vi "SQLite-Modes.vi"   [LabVIEW 2020]
uses:
  <vilib>/drjdpowell/SQLite Library/SQL Statement/SQL Statement.lvclass/SQL Statement.ctl
  <vilib>/drjdpowell/SQLite Library/SQL Connection/Open (path).vi
  <vilib>/drjdpowell/SQLite Library/SQL Statement/Bind Integer.vi
  <vilib>/drjdpowell/SQLite Library/SQL Statement/Bind Real.vi
  <vilib>/drjdpowell/SQLite Library/SQL Statement/Bind Text.vi
  <vilib>/drjdpowell/SQLite Library/SQL Connection/Open (string).vi
  <vilib>/drjdpowell/SQLite Library/SQL Statement/Step.vi
  <vilib>/AdvancedString/Path To Command Line String.vi
  <vilib>/drjdpowell/SQLite Library/SQL Connection/Execute SQL (No results).vi
  <vilib>/drjdpowell/SQLite Library/SQL Statement/Error Message.vi
  <vilib>/drjdpowell/SQLite Library/SQL Connection/Connection.lvclass
  <vilib>/drjdpowell/SQLite Library/SQL Statement/SQL Statement.lvclass
  <vilib>/drjdpowell/SQLite Library/SQLite.lvlib
  <vilib>/drjdpowell/SQLite Library/Transaction Helpers/Transaction.lvlib
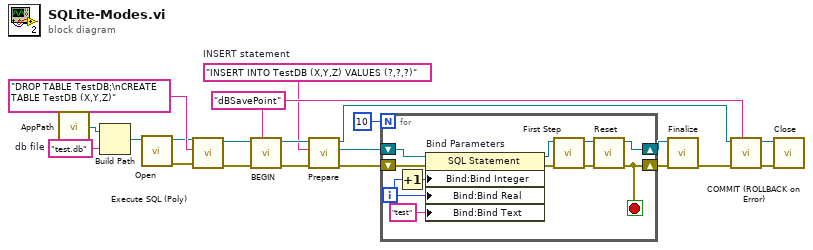
[diagram p0: block diagram]
diagram:
  w14 = "dBSavePoint" ("Savepoint name")
  w9 = "INSERT INTO TestDB (X,Y,Z) VALUES (?,?,?)"  # INSERT statement
  w19 = "test.db"  # db file
  n1 = call "AppPath.vi"() -> ("AppPath"=w1:path)
  n2 = Build Path(base path=w1, name or relative path=w19) -> (appended path=w17:path)
  n3 = call-poly <vilib>:"Open.vi"("db file"=w17) -> ("error out"=w18:errorcluster, "SQLite Connection"=w20:refnum<class "Connection.lvclass">)  [unwired: 9 in]
  n4 = call-poly <vilib>:"Execute SQL (Poly).vi"("error in (no error)"=w18, "SQL"="DROP TABLE TestDB;\nCREATE TABLE TestDB (X,Y,Z)", "SQLite Connection in"=w20) -> ("error out"=w5:errorcluster, "SQLite Connection"=w6:refnum<class "Connection.lvclass">)  [unwired: 7 in]
  n5 = call <vilib>:"BEGIN.vi"("Savepoint name"=w14, "error in (no error)"=w5, "SQLite Connection in"=w6) -> ("error out"=w13:errorcluster, "SQLite Connection"=w12:refnum<class "Connection.lvclass">)  [unwired: 7 in]
  n6 = call <vilib>:"Prepare.vi"("error in (no error)"=w13, "SQL"=w9, "SQLite Connection in"=w12) -> ("error out"=w8:errorcluster, "SQL Statement"=w7:refnum<class "SQL Statement.lvclass">, "SQLite Connection"=w15:refnum<class "Connection.lvclass">)  [unwired: 4 in, 2 out]
  n7 = for "For each set of parameters to be inserted..." {
    N: 10 -> [_]
    shift-right: [w26] -> w10
    shift-left: w7 -> [w32]
    shift-right: [w25] -> w11
    shift-left: w8 -> [w29]
    i -> [w23]
    stop <- w25 stop-if-true
    n8 = Increment(x=w23) -> (x+1=w24:i32)
    n9 = property on="Bind Parameters" class="SQL Statement"(reference=w32, error in=w29, "Bind:Bind Integer"=w24, "Bind:Bind Real"=w23, "Bind:Bind Text"="test" ("Bind:Text")) -> (reference out=w31:refnum<class "SQL Statement.lvclass">, error out=w30:errorcluster)
    n10 = call <vilib>:"First Step.vi"("error in (no error)"=w30, "SQL Statement in"=w31) -> ("error out"=w28:errorcluster, "SQL Statement"=w27:refnum<class "SQL Statement.lvclass">)  [unwired: 7 in, 1 out]
    n11 = call <vilib>:"Reset.vi"("error in (no error)"=w28, "SQL Statement in"=w27) -> ("error out"=w25:errorcluster, "SQL Statement"=w26:refnum<class "SQL Statement.lvclass">)  [unwired: 8 in]
  }
  n12 = call <vilib>:"Finalize.vi"("error in (no error)"=w11, "SQL Statement in"=w10) -> ("error out"=w16:errorcluster)  [unwired: 9 in]
  n13 = call <vilib>:"COMMIT (ROLLBACK on Error).vi"("Savepoint name"=w14, "error in (no error)"=w16, "SQLite Connection in"=w15) -> ("error out"=w3:errorcluster, "SQLite Connection"=w2:refnum<class "Connection.lvclass">)  [unwired: 7 in]
  n14 = call-dynamic "Close.vi"("error in (no error)"=w3, "SQLite Connection in"=w2) -> ()  [unwired: 9 in, 1 out]
